vi "UPH Panel.vi"(8 "error in (no error)":errorcluster, 10 "Base path":path=path "D:/Inalfa_Work/Project Program/FTT_Project/TP3_FTT/system", 11 "UPH in":T1[](array[typedef])) -> (0 "error out":errorcluster, 3 "UPH out":T1[](array[typedef]))   [LabVIEW 2014]
uses:
  Type'def/UPH Config.ctl
panel:
  in  "Cancel":bool
  in  "Save":bool
  in  "UPH":T1[](array[typedef])
  # "UPH Config"
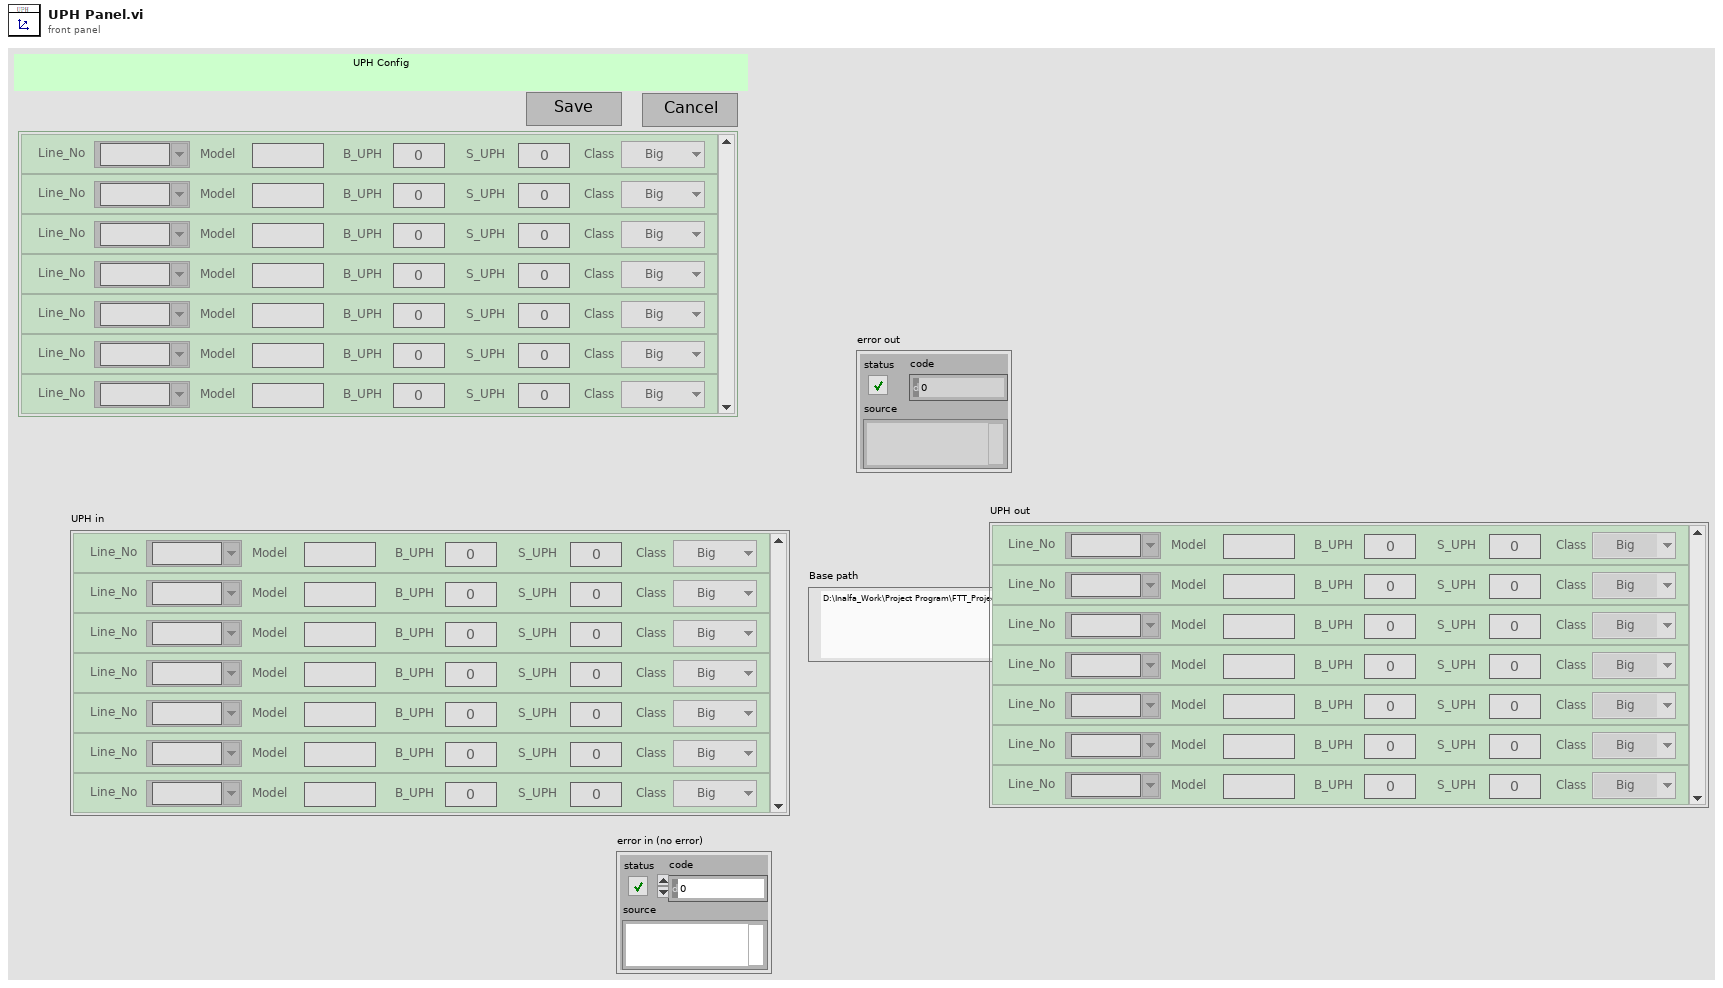
[diagram p1: front panel]
types:
  T1 = typedef "UPH Config.ctl" = cluster{"Line_No":string, "Model":string, "B_UPH ":i16, "S_UPH  ":i16, "Class":enum16{"Big", "Small"}}
  T2 = cluster{"UPH in":T1[], "Base path":path, "UPH":refnum<vi>}
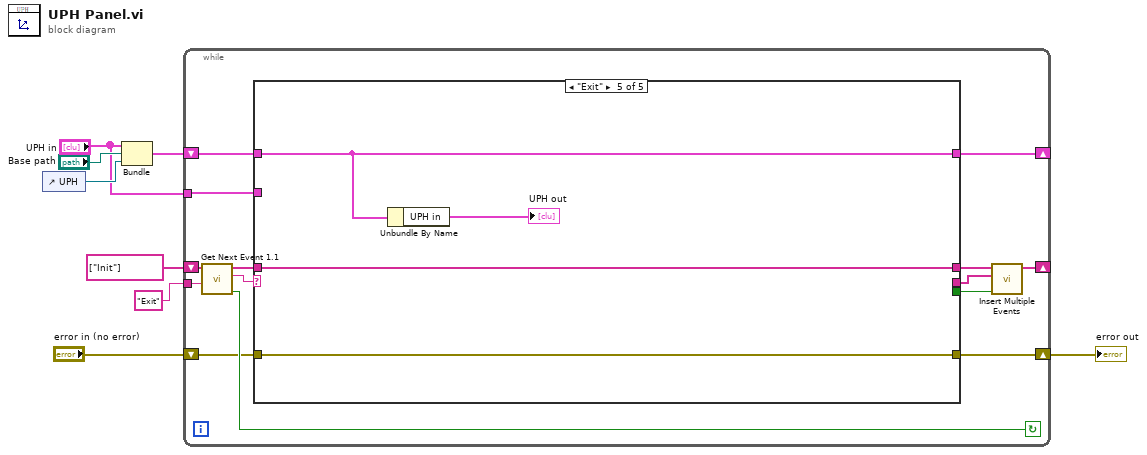
[diagram p0: block diagram]
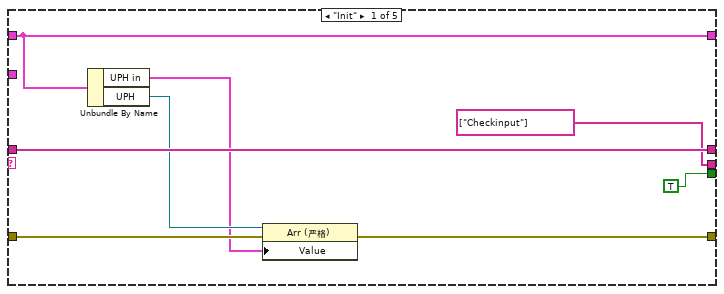
[diagram p2: hidden frame]
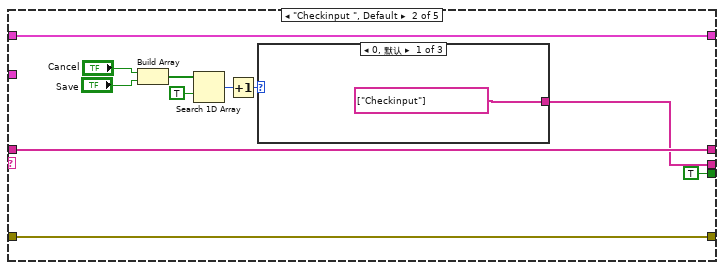
[diagram p3: hidden frame]
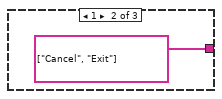
[diagram p4: hidden frame]
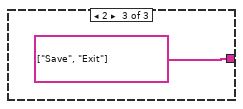
[diagram p5: hidden frame]
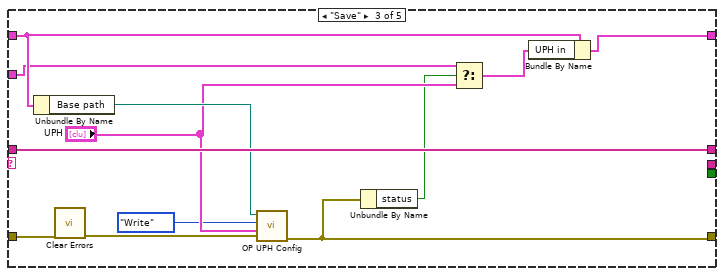
[diagram p6: hidden frame]
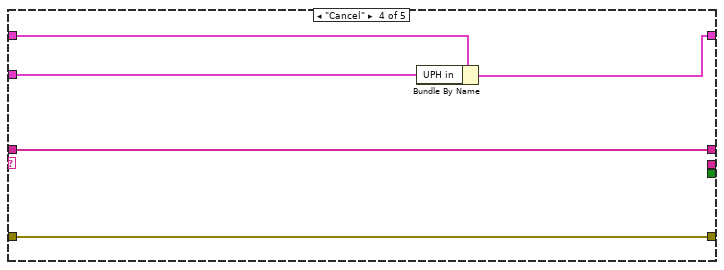
[diagram p7: hidden frame]
diagram:
  n1 = control-ref of="UPH"() -> (w6:refnum<vi>)
  n2 = Bundle("UPH in"="UPH in", "Base path"="Base path", "UPH"=w6) -> (w5:T2)  [unwired: 1 in]
  n3 = while {
    shift-right: [w16] -> _
    shift-left: string[] ["Init"] ("event queue in") -> [w20]
    shift-right: [w10] -> _
    shift-left: w5 -> [w11]
    tunnel: "Exit" -> [w19]
    tunnel: "UPH in" -> [w9]
    shift-right: [w12] -> w2
    shift-left: "error in (no error)" -> [w18]
    stop <- w21 continue-if-true
    n4 = call "Get Next Event 1.1.vi"("Exit Event"=w19, "event queue in"=w20) -> ("Condition (Exit:F)"=w21:bool, "next event"=w22:string, "event queue out"=w17:string[])  [unwired: 6 in, 1 out]
    n5 = case shown="\"Exit\"" w22 {
      tunnel: w18 -> [w27 w40 w46 w57 w64]
      tunnel: w17 -> [w30 w41 w56 w58 w63]
      tunnel: [w30 w41 w56 w58 w63] -> w15
      tunnel: [TRUE TRUE _ _ _] -> w14
      tunnel: [string[] ["Checkinput"] w34 _ _ _] -> w13
      tunnel: [w24 w40 w48 w57 w64] -> w12
      tunnel: w11 -> [w23 w39 w55 w61 w65]
      tunnel: [w23 w39 w53 w59 w65] -> w10
      tunnel: w9 -> [_ _ w52 w60 _]
      frame "Init" {
        n6 = Unbundle By Name(w23) -> ("UPH in"=w25:T1[], "UPH"=w26:refnum<vi>)
        n7 = property class="Arr (严格)"(reference=w26, error in=w27, "Value"=w25) -> (error out=w24:errorcluster)  [unwired: 1 out]
      }
      frame "Checkinput ", Default {
        n8 = Build Array("Cancel", "Save") -> (w36:bool[])
        n9 = Search 1D Array(1D array=w36, element=TRUE) -> (index of element=w32:i32)  [unwired: 1 in]
        n10 = Increment(x=w32) -> (x+1=w31:i32)
        n11 = case shown="0, 默认" w31 {
          tunnel: [string[] ["Checkinput"] string[] ["Cancel", "Exit"] string[] ["Save", "Exit"]] -> w34
          frame 0, Default {
          }
          frame 1 {
          }
          frame 2 {
          }
        }
      }
      frame "Save" {
        n12 = Unbundle By Name(w55) -> ("Base path"=w51:path)
        n13 = call <vilib>:"Clear Errors.vi"("error in (no error)"=w46) -> ("error out"=w45:errorcluster)  [unwired: 5 in, 1 out]
        n14 = call "OP UPH Config.vi"("error in (no error)"=w45, "UPH"="UPH", "Enum"=enum16{"init", "Read", "Write"}."Write", "Path"=w51) -> ("error out"=w48:errorcluster)  [unwired: 5 in, 2 out]
        n15 = Unbundle By Name(w48) -> ("status"=w47:bool)
        n16 = Select(t=w52, s=w47, f="UPH") -> (s? t:f=w54:T1[])
        n17 = Bundle By Name(cluster=w55, "UPH in"=w54) -> (w53:T2)
      }
      frame "Cancel" {
        n18 = Bundle By Name(cluster=w61, "UPH in"=w60) -> (w59:T2)
      }
      frame "Exit" {
        n19 = Unbundle By Name(w65) -> ("UPH in"=→"UPH out":T1[])
      }
    }
    n20 = call "Insert Multiple Events.vi"("Insert all? (T)"=w14, "Events to Insert"=w13, "Event queue in"=w15) -> ("Event queue out"=w16:string[])  [unwired: 4 in]
  }
  "error out" <- w2
